vi "circuits-capacitor.vi"(1 "Invert Y":bool, 2 "Invert X":bool, 4 "L2":dbl=0.05, 5 "L3":dbl=0.5, 6 "Swap-XY":bool, 7 "L1":dbl=0.1, 8 "Device in Y":refnum<k24>, 9 "GetPOS Y":refnum<vi>, 10 "GetPOS X":refnum<vi>, 11 "Device in X":refnum<k24>) -> (0 "Device out Y":refnum<k24>, 3 "Device out X":refnum<k24>)   [LabVIEW 2014]
doc: "André Romero - 2019\nandretec@ifsc.usp.br"
uses:
  C:/user-Lab/AndreTec/GITs/andretec/Thorlabs-Vector-Move/kinesisTec/Kinesis/Thorlabs.MotionControl.TCube.DCServoCLI.dll
  kinesisTec/Kinesis/Thorlabs.MotionControl.TCube.DCServoCLI.dll
panel:
  out "-x":dbl=-0.5
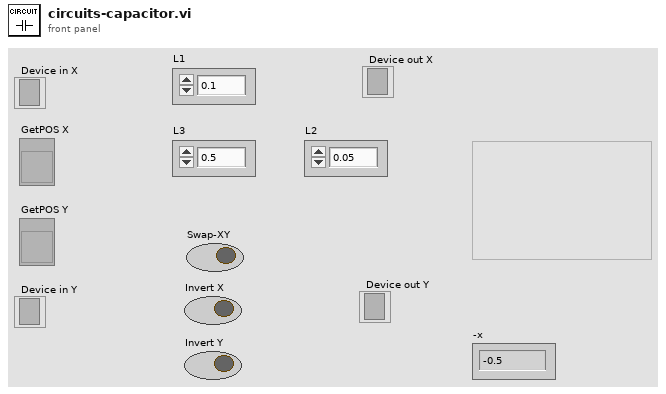
[diagram p1: front panel]
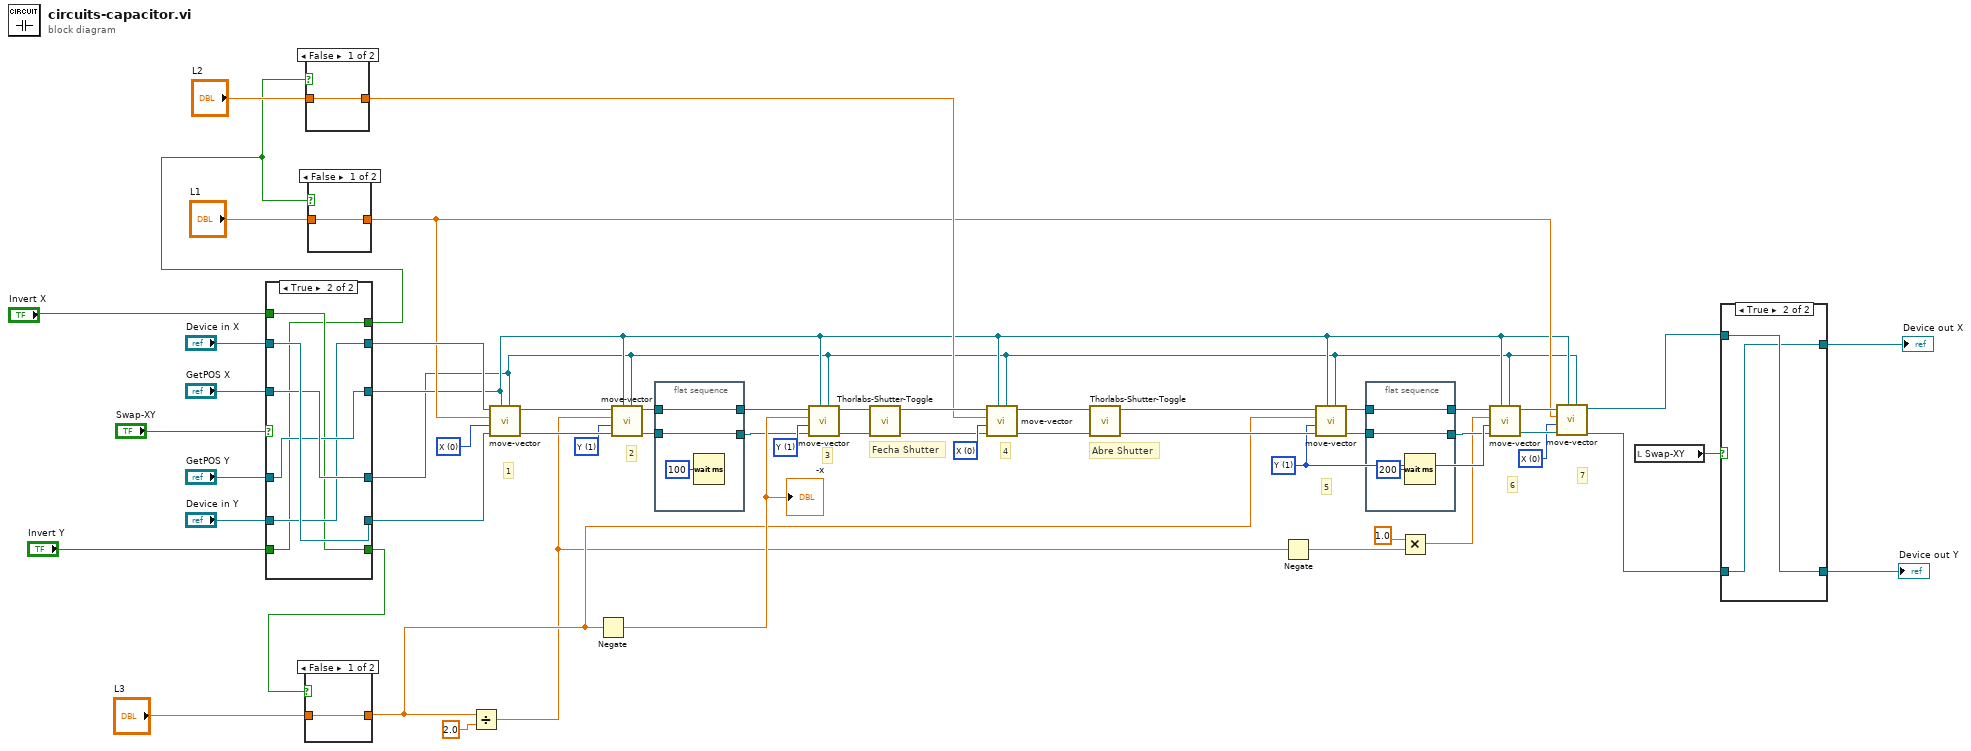
[diagram p0: block diagram]
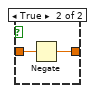
[diagram p3: hidden frame]
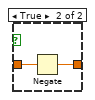
[diagram p4: hidden frame]
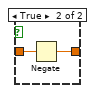
[diagram p5: hidden frame]
diagram:
  w20 = u16 1 items=["X", "Y"] ("X-Y")
  w23 = u16 0 items=["X", "Y"] ("X-Y")
  w29 = u16 1 items=["X", "Y"] ("X-Y")
  w43 = u16 0 items=["X", "Y"] ("X-Y")
  w37 = u16 1 items=["X", "Y"] ("X-Y")
  w47 = u16 0 items=["X", "Y"] ("X-Y")
  # "7"
  # "6"
  # "5"
  # "4"
  # "3"
  # "2"
  # "1"
  # "Abre Shutter"
  # "Fecha Shutter"
  n1 = case shown="True" "Swap-XY" {
    tunnel: "Device in X" -> [w60 w68]
    tunnel: [w60 w65] -> w49
    tunnel: "GetPOS Y" -> [w62 w66]
    tunnel: [w62 w67] -> w21
    tunnel: "Device in Y" -> [w61 w65]
    tunnel: [w61 w68] -> w48
    tunnel: "GetPOS X" -> [w59 w67]
    tunnel: [w59 w66] -> w22
    tunnel: "Invert X" -> [w58 w64]
    tunnel: [w58 w63] -> w10
    tunnel: "Invert Y" -> [w57 w63]
    tunnel: [w57 w64] -> w8
    frame False {
    }
    frame True {
    }
  }
  n2 = case shown="False" w8 {
    tunnel: "L3" -> [w69 w71]
    tunnel: [w69 w70] -> w30
    frame False {
    }
    frame True {
      n3 = Negate(x=w71) -> (-x=w70:dbl)
    }
  }
  n4 = case shown="False" w10 {
    tunnel: "L2" -> [w72 w74]
    tunnel: [w72 w73] -> w31
    frame False {
    }
    frame True {
      n5 = Negate(x=w74) -> (-x=w73:dbl)
    }
  }
  n6 = case shown="False" w10 {
    tunnel: "L1" -> [w75 w77]
    tunnel: [w75 w76] -> w24
    frame False {
    }
    frame True {
      n7 = Negate(x=w77) -> (-x=w76:dbl)
    }
  }
  n8 = Divide(x=w30, y=2.0) -> (x/y=w28:dbl)
  n9 = call "move-vector.vi"("GetPOS Y"=w21, "GetPOS X"=w22, "Device in Y"=w48, "X-Y"=w47, "Distance"=w24, "Device in X"=w49) -> ("Device out Y"=w45:refnum<k24>, "Device out X"=w46:refnum<k24>)  [unwired: 4 in]
  n10 = Negate(x=w30) -> (-x=w34:dbl)
  "-x" <- w34
  n11 = call "move-vector.vi"("GetPOS Y"=w21, "GetPOS X"=w22, "Device in Y"=w45, "X-Y"=w37, "Distance"=w28, "Device in X"=w46) -> ("Device out Y"=w17:refnum<k24>, "Device out X"=w19:refnum<k24>)  [unwired: 4 in]
  n12 = flat-sequence {
    tunnel: [w80] -> w18
    tunnel: w19 -> [w80]
    tunnel: w17 -> [w79]
    tunnel: [w79] -> w16
    frame #0 {
      n13 = Wait (ms)(milliseconds to wait=u32 100) -> ()  [unwired: 1 out]
    }
  }
  n14 = call "move-vector.vi"("GetPOS Y"=w21, "GetPOS X"=w22, "Device in Y"=w16, "X-Y"=w20, "Distance"=w34, "Device in X"=w18) -> ("Device out Y"=w35:refnum<k24>, "Device out X"=w36:refnum<k24>)  [unwired: 4 in]
  n15 = call "Thorlabs-Shutter-Toggle.vi"("Device in Y"=w35, "Device in X"=w36) -> ("Device out Y"=w42:refnum<k24>, "Device out X"=w44:refnum<k24>)  [unwired: 8 in]
  n16 = call "move-vector.vi"("GetPOS Y"=w21, "GetPOS X"=w22, "Device in Y"=w42, "X-Y"=w43, "Distance"=w31, "Device in X"=w44) -> ("Device out Y"=w40:refnum<k24>, "Device out X"=w41:refnum<k24>)  [unwired: 4 in]
  n17 = call "Thorlabs-Shutter-Toggle.vi"("Device in Y"=w40, "Device in X"=w41) -> ("Device out Y"=w38:refnum<k24>, "Device out X"=w39:refnum<k24>)  [unwired: 8 in]
  n18 = Negate(x=w28) -> (-x=w27:dbl)
  n19 = call "move-vector.vi"("GetPOS Y"=w21, "GetPOS X"=w22, "Device in Y"=w38, "X-Y"=w29, "Distance"=w30, "Device in X"=w39) -> ("Device out Y"=w14:refnum<k24>, "Device out X"=w15:refnum<k24>)  [unwired: 4 in]
  n20 = flat-sequence {
    tunnel: [w83] -> w13
    tunnel: w15 -> [w83]
    tunnel: w14 -> [w82]
    tunnel: [w82] -> w12
    frame #0 {
      n21 = Wait (ms)(milliseconds to wait=u32 200) -> ()  [unwired: 1 out]
    }
  }
  n22 = Multiply(x=1.0, y=w27) -> (x*y=w2:dbl)
  n23 = call "move-vector.vi"("GetPOS Y"=w21, "GetPOS X"=w22, "Device in Y"=w12, "X-Y"=w29, "Distance"=w2, "Device in X"=w13) -> ("Device out Y"=w25:refnum<k24>, "Device out X"=w26:refnum<k24>)  [unwired: 4 in]
  n24 = call "move-vector.vi"("GetPOS Y"=w21, "GetPOS X"=w22, "Device in Y"=w25, "X-Y"=w23, "Distance"=w24, "Device in X"=w26) -> ("Device out Y"=w5:refnum<k24>, "Device out X"=w6:refnum<k24>)  [unwired: 4 in]
  n25 = local read "Swap-XY"() -> (w7:bool)
  n26 = case shown="True" w7 {
    tunnel: w6 -> [w85 w87]
    tunnel: [w85 w86] -> w4
    tunnel: w5 -> [w84 w86]
    tunnel: [w84 w87] -> w3
    frame False {
    }
    frame True {
    }
  }
  "Device out X" <- w4
  "Device out Y" <- w3
